vi "RDS Serial Init Port.vi"(8 "error in (no error)":errorcluster, 11 "RDS Serial Instrument Actor in":refnum<class "RDS Serial Instrument Actor.lvclass">) -> (0 "error out":errorcluster, 3 "RDS Serial Instrument Actor out":refnum<class "RDS Serial Instrument Actor.lvclass">)   [LabVIEW 2015, in "RDS Abstracts.lvlib" / "RDS Serial Instrument Actor.lvlib" / "RDS Serial Instrument Actor.lvclass"]
uses:
  RDS Serial Instrument Actor.lvclass
  RDS Serial Instrument Actor.lvclass/RDS Serial Instrument Actor.ctl
  Libraries/RDS Serial Handler/RDS Serial Instrument.lvclass
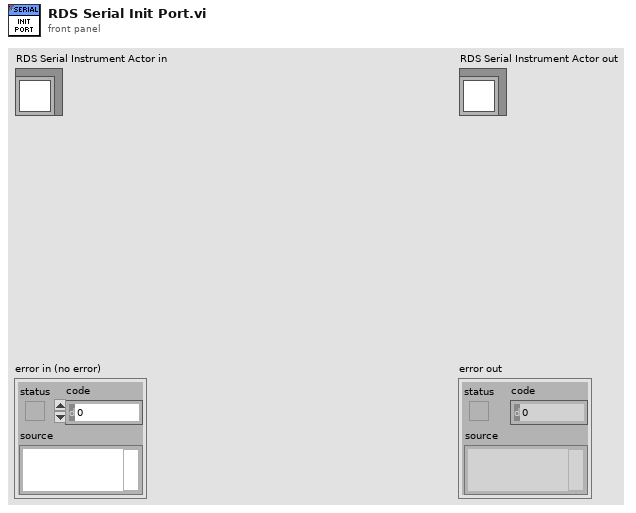
[diagram p1: front panel]
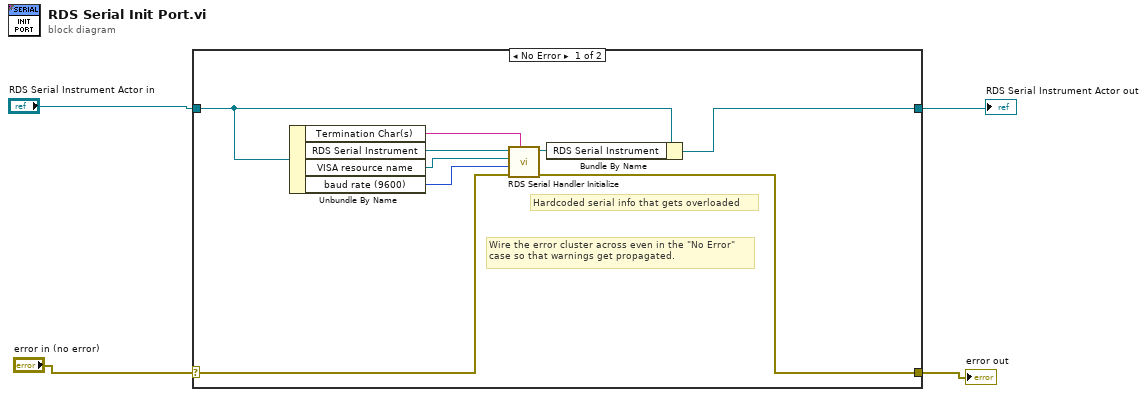
[diagram p0: block diagram]
diagram:
  n1 = case shown="No Error" "error in (no error)" {
    selector: "error in (no error)" -> [w6 w15]
    tunnel: [w5 w15] -> w2
    tunnel: [w11 w14] -> w1
    tunnel: "RDS Serial Instrument Actor in" -> [w10 w14]
    frame No Error {
      # "Hardcoded serial info that gets overloaded"
      # "Wire the error cluster across even in the \"No Error\"\ncase so that warnings get propagated."
      n2 = Unbundle By Name(w10) -> ("Termination Char(s)"=w9:string, "RDS Serial Instrument"=w13:refnum<class "RDS Serial Instrument.lvclass">, "VISA resource name"=w8:refnum<visa-resource-name>, "baud rate (9600)"=w7:u32)
      n3 = call "RDS Serial Handler Initialize.vi"("Termination Char(s)"=w9, "error in (no error)"=w6, "baud rate (9600)"=w7, "VISA resource name"=w8, "RDS Serial Instrument in"=w13) -> ("error out"=w5:errorcluster, "RDS Serial Instrument out"=w12:refnum<class "RDS Serial Instrument.lvclass">)  [unwired: 5 in]
      n4 = Bundle By Name(cluster=w10, "RDS Serial Instrument"=w12) -> (w11:refnum<class "RDS Serial Instrument Actor.lvclass">)
    }
    frame Error {
    }
  }
  "error out" <- w2
  "RDS Serial Instrument Actor out" <- w1
